vi "File.Delete Dir if is Empty.vi"(8 "error in (no error)":errorcluster, 10 "Delete if is Empty":bool, 11 "Dir":path) -> (0 "error out":errorcluster, 1 "Folders":i32, 2 "Files":i32, 3 "Empty":bool)   [LabVIEW 2019]
uses:
  <vilib>/KATE/Files/File Utils.lvlib
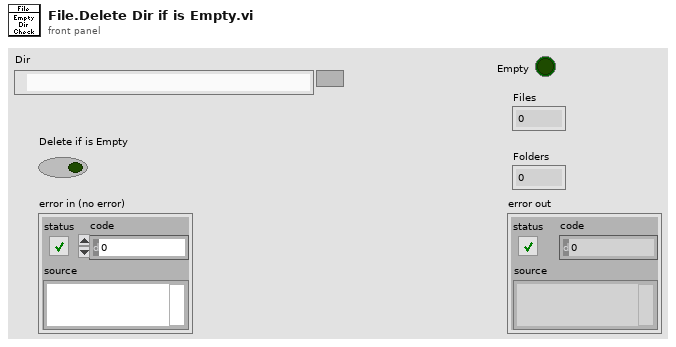
[diagram p1: front panel]
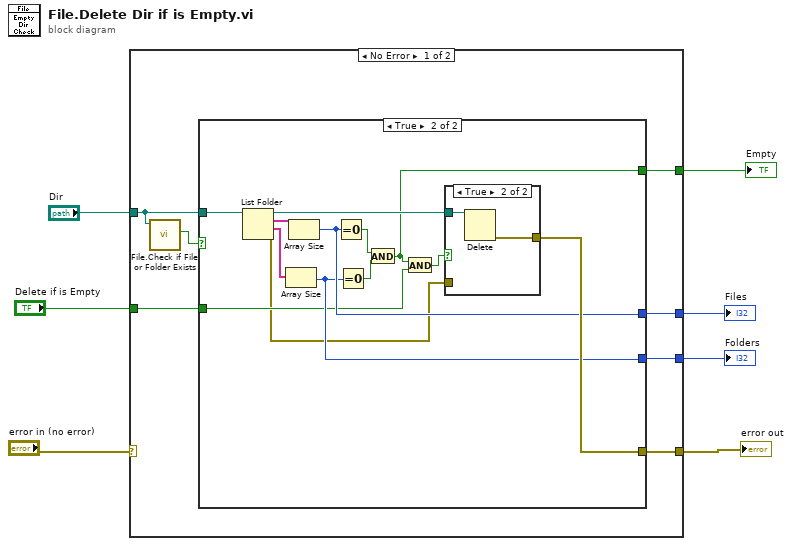
[diagram p0: block diagram]
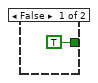
[diagram p2: hidden frame]
diagram:
  n1 = case shown="No Error" "error in (no error)" {
    selector: "error in (no error)" -> [_ w31]
    tunnel: "Dir" -> [w9 _]
    tunnel: [w14 w31] -> w5
    tunnel: [w11 _] -> w4
    tunnel: [w13 _] -> w3
    tunnel: [w12 _] -> w2
    tunnel: "Delete if is Empty" -> [w10 _]
    frame No Error {
      n2 = call <vilib>:"File.Check if File or Folder Exists.vi"("Path"=w9) -> ("Exists"=w8:bool)  [unwired: 6 in, 4 out]
      n3 = case shown="True" w8 {
        tunnel: w9 -> [_ w28]
        tunnel: [_ w22] -> w14
        tunnel: [_ w21] -> w13
        tunnel: [_ w20] -> w12
        tunnel: [TRUE w19] -> w11
        tunnel: w10 -> [_ w17]
        frame False {
        }
        frame True {
          n4 = List Folder(path=w28) -> (path out=w23:path, filenames=w27:string[], folder names=w26:string[], error out=w16:errorcluster)  [unwired: 3 in]
          n5 = Array Size(array=w26) -> (size(s)=w20:i32)
          n6 = Array Size(array=w27) -> (size(s)=w21:i32)
          n7 = Equal To 0?(x=w21) -> (x = 0?=w24:bool)
          n8 = Equal To 0?(x=w20) -> (x = 0?=w25:bool)
          n9 = And(x=w24, y=w25) -> (x .and. y?=w19:bool)
          n10 = And(x=w19, y=w17) -> (x .and. y?=w18:bool)
          n11 = case shown="True" w18 {
            tunnel: w23 -> [_ w30]
            tunnel: [_ w29] -> w22
            tunnel: w16 -> [_ _]
            frame False {
            }
            frame True {
              n12 = Delete(path (use dialog)=w30) -> (error out=w29:errorcluster)  [unwired: 4 in, 2 out]
            }
          }
        }
      }
    }
    frame Error {
    }
  }
  "Empty" <- w4
  "error out" <- w5
  "Files" <- w3
  "Folders" <- w2
